vi "Script Request and Wait For Reply Custom Timeout.vi"(8 "error in":errorcluster, 10 "VI Ref":refnum<vi>, 11 "Theme":bool) -> (0 "error out":errorcluster)   [LabVIEW 2019, in "Panther Dashboard.lvlib"]
uses:
  Panther Dashboard.lvlib
  <vilib>/Utility/traverseref.llb/TRef TravTarget.ctl
  Panther Dashboard--global.vi
panel:
  in  "Continue":bool
  in  "Cancel":bool
  in  "Custom Timeout for Request and Wait for Reply":i32 format="%d ms"
  # "- The 'Module Timeout--constant.vi' in the DQMH Framework serves as a mechanism to control the maximum time a 'Request and Wait for Reply' waits for a response.\n- By default, this timeout value is set to 5000 milliseconds (ms), which translates to 5 seconds.\n\n**When to Use Custom Timeout for a Request and Wait for Reply:**\n\n- Consider altering the Timeout value for a Request and Wait for Reply in the following scenarios:\n    - If a module is inherently slow-responding to a specific Request and Wait for reply due to complex calculations or external interactions, you might need to increase the Timeout to prevent premature timeouts.\n    - Conversely, if you're confident that a module's response  to a specifig Request and Wait for Reply should typically be much faster than 5 seconds, you could decrease the Timeout to optimize performance and avoid unnecessary waiting.\n\nExample:\n-You have a Connect to Hardware Request and Wait for Reply Event.\n-This request transmits the COM port information to the hardware module.\n-In return, you anticipate receiving a response containing the hardware ID (HW ID) as the payload (data).\n-You're confident that if the hardware is connected and functioning correctly, a response should be received within a maximum of 100 milliseconds (ms).\n-Based on your certainty about the expected response time, you've opted to establish a custom timeout value of 200 ms.\nThis signifies that the Request and Wait for Reply operation will only wait for a maximum of 200 ms for the hardware's response before getting a timeout error.\n\nNOTES:\n\n- Exercise caution when reducing the timeout excessively, as it could lead to premature timeouts and disrupt your application's functionality.\n\nUse Restore to Module's Timeout to undo this action."
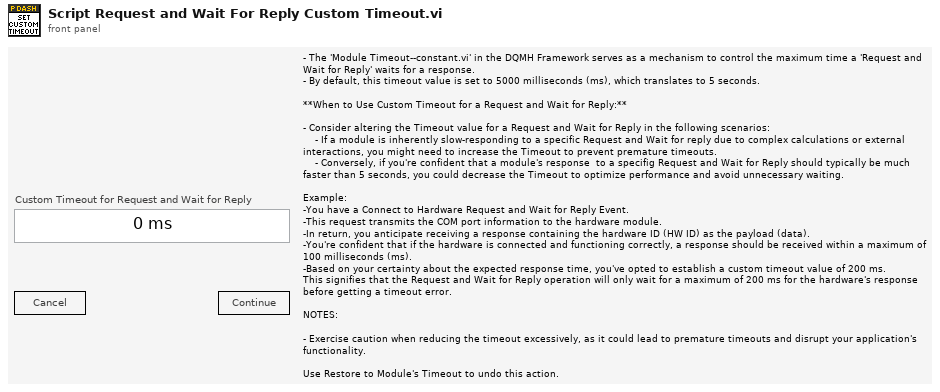
[diagram p1: front panel]
types:
  T1 = typedef "TRef TravTarget.ctl" = enum16{"FP", "BD", "Other"}
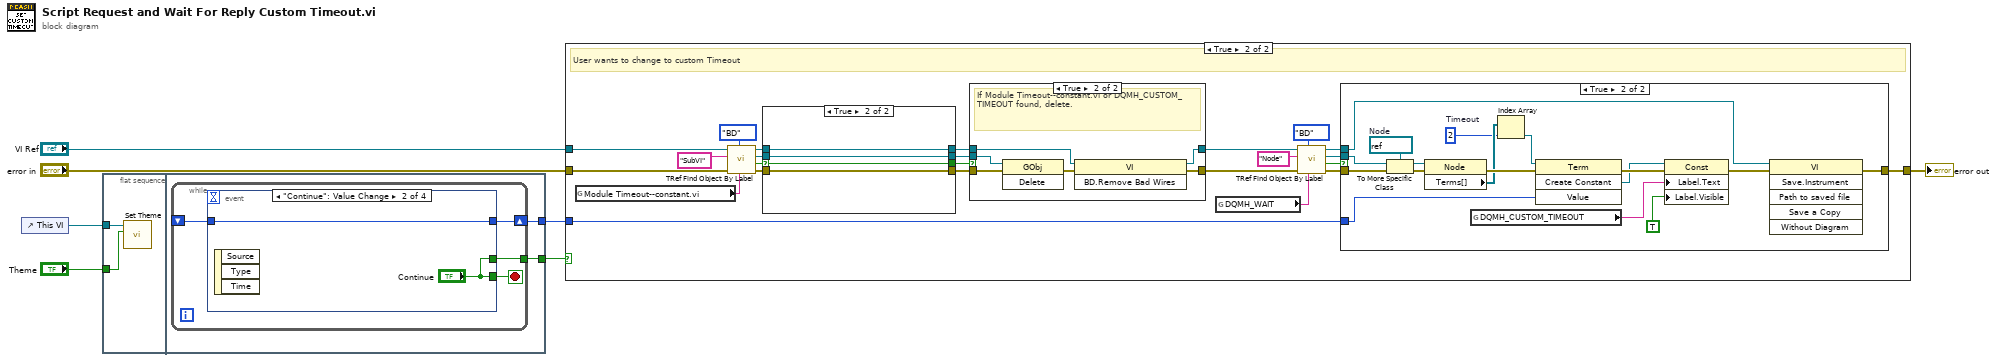
[diagram p0: block diagram]
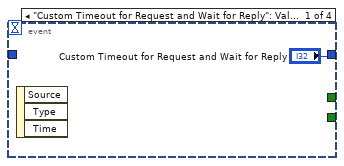
[diagram p2: hidden frame]
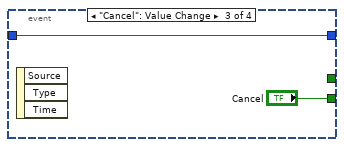
[diagram p3: hidden frame]
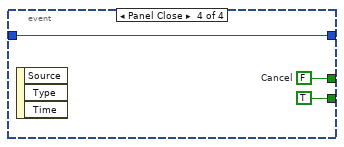
[diagram p4: hidden frame]
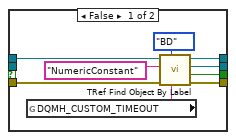
[diagram p8: hidden frame]
diagram:
  n1 = control-ref of="This VI"() -> (w2:refnum<vi>)
  n2 = flat-sequence {
    tunnel: w2 -> [w9]
    tunnel: "Theme" -> [w8]
    tunnel: [w11] -> w4
    tunnel: [w10] -> w3
    frame #0 {
      n3 = call "Set Theme.vi"("Dark?"=w8, "VI in"=w9) -> ()  [unwired: 10 in]
    }
    frame #1 {
      n4 = while {
        tunnel: [w14] -> w10
        shift-right: [w15] -> w11
        shift-left: _ -> [w12]
        stop <- w13 stop-if-true
        n5 = event shown="[1] \"Continue\": Value Change" {
          selector: _ -> [_ _ _ _]
          dyn-events: _ -> [_ _ _ _]
          timeout: _ -> [_ _ _ _]
          tunnel: ["Custom Timeout for Request and Wait for Reply" w18 w19 w22] -> w15
          tunnel: [_ "Continue" _ w21] -> w14
          tunnel: [_ "Continue" "Cancel" TRUE ("Cancel")] -> w13
          tunnel: w12 -> [_ w18 w19 w22]
          event "Custom Timeout for Request and Wait for Reply": Value Change {
            n6 = event-data() -> ()  [unwired: 1 in, 3 out]
          }
          event "Continue": Value Change {
            n7 = event-data() -> ()  [unwired: 1 in, 3 out]
          }
          event "Cancel": Value Change {
            n8 = event-data() -> ()  [unwired: 1 in, 3 out]
          }
          event Panel Close {
            w21 = FALSE  # Cancel
            n9 = event-data() -> ()  [unwired: 1 in, 3 out]
          }
        }
      }
    }
  }
  n10 = case shown="True" w3 {
    tunnel: [w24 w48] -> w7
    tunnel: "error in" -> [w24 w47]
    tunnel: "VI Ref" -> [_ w40]
    tunnel: w4 -> [_ w39]
    frame False {
      # "User Cancel"
    }
    frame True {
      # "User wants to change to custom Timeout"
      n11 = global read "Panther Dashboard--global.vi" "Module Timeout--constant.vi"() -> (w26:string)
      n12 = call <vilib>:"TRef Find Object By Label.vi"("Label"=w26, "Traverse Target"=TRef_TravTarget."BD", "error in (no error)"=w47, "Class Name"="SubVI", "VI Ref"=w40) -> ("error out"=w44:errorcluster, "Found?"=w28:bool, "Found Obj Ref"=w33:refnum<vi>, "dup VI Ref"=w31:refnum<vi>)  [unwired: 3 in]
      n13 = case shown="True" w28 {
        selector: w28 -> [_ w85]
        tunnel: w33 -> [_ w84]
        tunnel: [w77 w84] -> w32
        tunnel: w44 -> [w83 w87]
        tunnel: [w82 w87] -> w43
        tunnel: w31 -> [w79 w86]
        tunnel: [w78 w86] -> w30
        tunnel: [w76 w85] -> w27
        frame False {
          n14 = global read "Panther Dashboard--global.vi" "DQMH_CUSTOM_TIMEOUT"() -> (w75:string)
          n15 = call <vilib>:"TRef Find Object By Label.vi"("Label"=w75, "Traverse Target"=TRef_TravTarget."BD", "error in (no error)"=w83, "Class Name"="NumericConstant", "VI Ref"=w79) -> ("error out"=w82:errorcluster, "Found?"=w76:bool, "Found Obj Ref"=w77:refnum<vi>, "dup VI Ref"=w78:refnum<vi>)  [unwired: 3 in]
        }
        frame True {
        }
      }
      n16 = case shown="True" w27 {
        tunnel: [w50 w56] -> w45
        tunnel: w43 -> [w50 w54]
        tunnel: [w49 w53] -> w34
        tunnel: w32 -> [_ w52]
        tunnel: w30 -> [w49 w51]
        frame False {
        }
        frame True {
          # "If Module Timeout--constant.vi or DQMH_CUSTOM_TIMEOUT found, delete."
          n17 = invoke class="GObj" method="Delete"(reference=w52, error in=w54) -> (error out=w55:errorcluster)  [unwired: 1 in, 2 out]
          n18 = invoke class="VI" method="BD.Remove Bad Wires"(reference=w51, error in=w55) -> (reference out=w53:refnum<vi>, error out=w56:errorcluster)  [unwired: 1 in, 1 out]
        }
      }
      n19 = global read "Panther Dashboard--global.vi" "DQMH_WAIT"() -> (w25:string)
      n20 = call <vilib>:"TRef Find Object By Label.vi"("Label"=w25, "Traverse Target"=TRef_TravTarget."BD", "error in (no error)"=w45, "Class Name"="Node", "VI Ref"=w34) -> ("error out"=w46:errorcluster, "Found?"=w36:bool, "Found Obj Ref"=w37:refnum<vi>, "dup VI Ref"=w29:refnum<vi>)  [unwired: 3 in]
      n21 = case shown="True" w36 {
        tunnel: w37 -> [_ w68]
        tunnel: w46 -> [w57 w74]
        tunnel: [w57 w69] -> w48
        tunnel: w39 -> [_ w62]
        tunnel: w29 -> [_ w59]
        frame False {
        }
        frame True {
          w64 = 2  # Timeout
          w67 = refnum<vi> refnum  # Node
          n22 = To More Specific Class(target class=w67, reference=w68, error in=w74) -> (specific class reference=w66:refnum<vi>, error out=w73:errorcluster)
          n23 = property class="Node"(reference=w66, error in=w73) -> (error out=w72:errorcluster, "Terms[]"=w65:refnum<vi>[])  [unwired: 1 out]
          n24 = global read "Panther Dashboard--global.vi" "DQMH_CUSTOM_TIMEOUT"() -> (w58:string)
          n25 = Index Array(array=w65, index=w64) -> (element=w63:refnum<vi>)
          n26 = invoke class="Term" method="Create Constant"(reference=w63, error in=w72, "Value"=w62) -> (error out=w71:errorcluster, "Create Constant"=w61:refnum<vi>)  [unwired: 1 in, 2 out]
          n27 = property class="Const"(reference=w61, error in=w71, "Label.Text"=w58, "Label.Visible"=TRUE) -> (error out=w70:errorcluster)  [unwired: 1 out]
          n28 = invoke class="VI" method="Save.Instrument"(reference=w59, error in=w70) -> (error out=w69:errorcluster)  [unwired: 4 in, 5 out]
        }
      }
    }
  }
  "error out" <- w7
